vi "ControlMotorGetDefinedPostion.vi"(10 "位置":T2) -> (2 "PosOut":cluster{"控制电机":T1, "位置":dbl}[](array[cluster]))   [LabVIEW 2018]
panel:
  # "获得修正之后的位置"
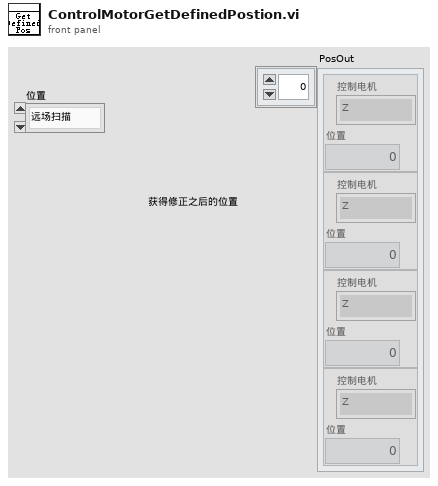
[diagram p1: front panel]
types:
  T1 = typedef "控制电机枚举器.ctl" = enum16{"Z", "Y", "X", "发散角", "俯仰", "旋转"}
  T2 = typedef "控制电机位置枚举器.ctl" = enum16{"远场扫描", "发散角扫描", "远场相机", "近场相机", "时间波形", "偏振", "能量", "功率", "光谱"}
  T3 = cluster{"远场相机":cluster{"控制电机":T1, "位置":dbl}[], "近场相机":cluster{"控制电机":T1, "位置":dbl}[], "时间波形":cluster{"控制电机":T1, "位置":dbl}[], "偏振":cluster{"控制电机":T1, "位置":dbl}[], "能量":cluster{"控制电机":T1, "位置":dbl}[], "功率":cluster{"控制电机":T1, "位置":dbl}[], "光谱":cluster{"控制电机":T1, "位置":dbl}[], "准直光焦点":cluster{"控制电机":T1, "位置":dbl}[]}
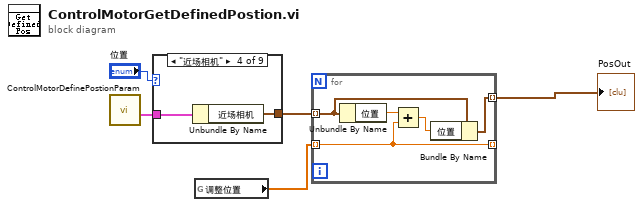
[diagram p0: block diagram]
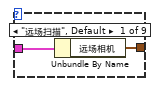
[diagram p2: hidden frame]
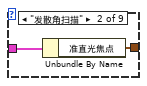
[diagram p3: hidden frame]
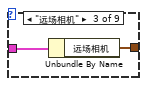
[diagram p4: hidden frame]
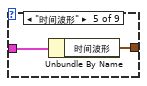
[diagram p5: hidden frame]
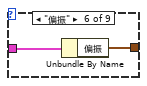
[diagram p6: hidden frame]
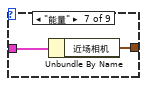
[diagram p7: hidden frame]
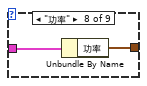
[diagram p8: hidden frame]
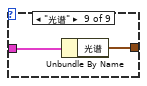
[diagram p9: hidden frame]
diagram:
  n1 = call "ControlMotorDefinePostionParam.vi"() -> ("位置信息"=w5:T3)  [unwired: 11 in]
  n2 = case shown="\"近场相机\"" "位置" {
    tunnel: w5 -> [w7 w9 w11 w13 w15 w17 w19 w21 w23]
    tunnel: [w6 w8 w10 w12 w14 w16 w18 w20 w22] -> w3
    frame "远场扫描", Default {
      n3 = Unbundle By Name(w7) -> ("远场相机"=w6:cluster{"控制电机":T1, "位置":dbl}[])
    }
    frame "发散角扫描" {
      n4 = Unbundle By Name(w9) -> ("准直光焦点"=w8:cluster{"控制电机":T1, "位置":dbl}[])
    }
    frame "远场相机" {
      n5 = Unbundle By Name(w11) -> ("远场相机"=w10:cluster{"控制电机":T1, "位置":dbl}[])
    }
    frame "近场相机" {
      n6 = Unbundle By Name(w13) -> ("近场相机"=w12:cluster{"控制电机":T1, "位置":dbl}[])
    }
    frame "时间波形" {
      n7 = Unbundle By Name(w15) -> ("时间波形"=w14:cluster{"控制电机":T1, "位置":dbl}[])
    }
    frame "偏振" {
      n8 = Unbundle By Name(w17) -> ("偏振"=w16:cluster{"控制电机":T1, "位置":dbl}[])
    }
    frame "能量" {
      n9 = Unbundle By Name(w19) -> ("近场相机"=w18:cluster{"控制电机":T1, "位置":dbl}[])
    }
    frame "功率" {
      n10 = Unbundle By Name(w21) -> ("功率"=w20:cluster{"控制电机":T1, "位置":dbl}[])
    }
    frame "光谱" {
      n11 = Unbundle By Name(w23) -> ("光谱"=w22:cluster{"控制电机":T1, "位置":dbl}[])
    }
  }
  n12 = global read "globalMessage.vi" "调整位置"() -> (w1:dbl[])
  n13 = for {
    tunnel: [w24] -> w2 mode=indexing
    tunnel: [w26] -> _ mode=indexing
    tunnel: w3 -> [w25] mode=indexing
    tunnel: w1 -> [w26] mode=indexing
    n14 = Unbundle By Name(w25) -> ("位置"=w28:dbl)
    n15 = Add(x=w28, y=w26) -> (x+y=w27:dbl)
    n16 = Bundle By Name(cluster=w25, "位置"=w27) -> (w24:cluster{"控制电机":T1, "位置":dbl})
  }
  "PosOut" <- w2
